vi "2-1.vi"(7 "kf(Hz/V)":dbl=50000.0, 8 "An(V)":dbl=0.02, 9 "带通Butterworth滤波器":cluster{"中心频率(Hz)":dbl, "带宽(Hz)":dbl}={"中心频率(Hz)"=150000.0, "带宽(Hz)"=220000.0}, 10 "调制信号":cluster{"fm(Hz)":dbl, "Am(V)":dbl}={"fm(Hz)"=5000.0, "Am(V)"=1.0}, 11 "载波信号":cluster{"fc(Hz)":dbl, "Ac(V)":dbl}={"fc(Hz)"=150000.0, "Ac(V)"=1.0}) -> (1 "频域":cluster{"f0":dbl, "df":dbl, "magnitude":dbl[]}(graph), 2 "时域 2":waveform(dbl)[](graph), 3 "时域":waveform(dbl)[](graph))   [LabVIEW 2018]
uses:
  <vilib>/Analysis/3filter.llb/Filter Passband Type.ctl
  <vilib>/Analysis/3filter.llb/Butterworth Filter (DBL).vi
  <vilib>/express/express analysis/Spectral/Block/exnSpectralBlock spectral measurements peak poly.vi
  <vilib>/express/express analysis/Spectral/Block/exnSpectralBlock spectral measurements peak WFM.vi
  <vilib>/express/express analysis/Spectral/XNode/ExpressSpectralMeasurementsBlockNode.xnode
  <vilib>/measure/NI_MABase.lvlib
  <vilib>/Analysis/NI_AALPro.lvlib
  <vilib>/Analysis/NI_AALBase.lvlib
panel:
  out "fh":dbl
  out "fl":dbl
  in  "选项卡控件":enum32{"调制", "滤波", "解调"}(tab)
  out "频域":cluster{"f0":dbl, "df":dbl, "magnitude":dbl[]}(graph)
  out "时域":waveform(dbl)(graph)
  out "卡森定则理论BT(Hz)":dbl
  out "数组":dbl[](array[numeric])
  out "调制信号":waveform(dbl)(graph)
  out "积分信号":waveform(dbl)(graph)
  out "采样参数（采样频率fs，采样数Ns）":cluster{dbl, dbl} {"?" format="%#_6f"; "?" format="%#_6f"}
  out "载波信号":waveform(dbl)(graph)
  # "采样率取1000*fc\n要显示n个周期的调制信号波形，\n则采样数Ns=n*fs/fm\nfh和fl为解调前滤波器\n的高和低截止频率"
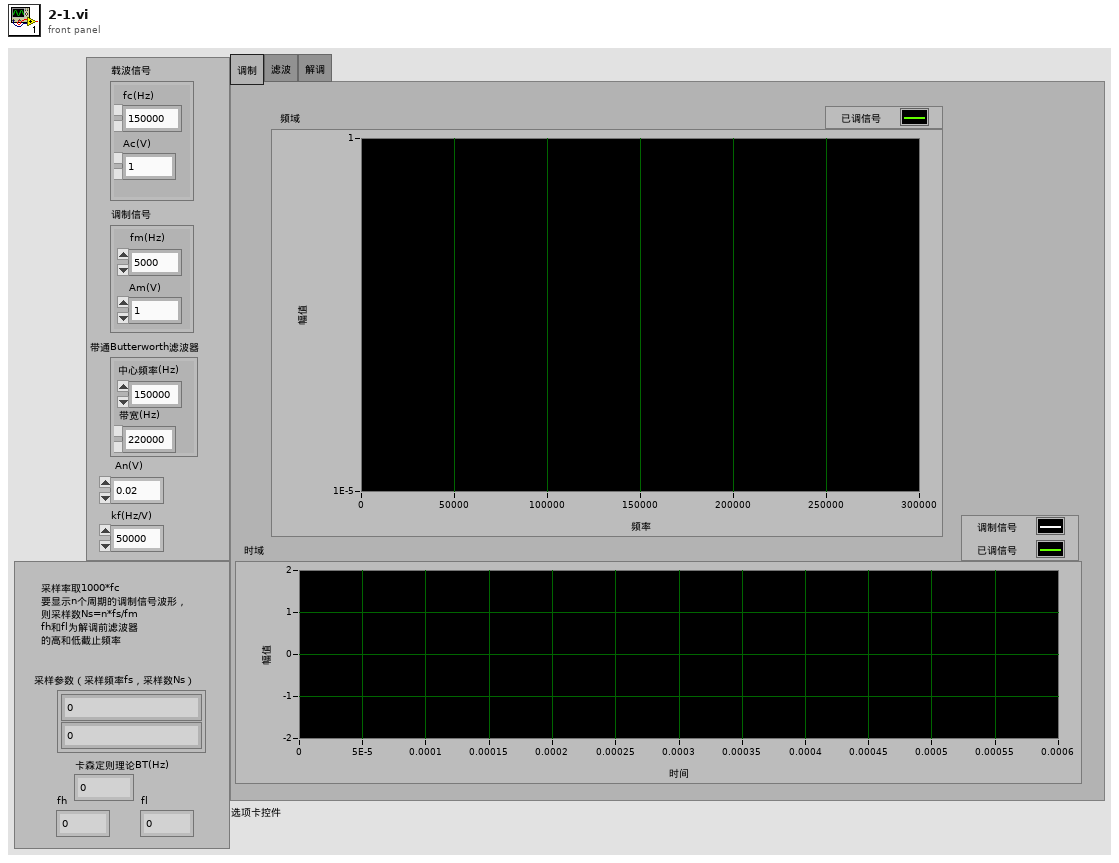
[diagram p1: front panel]
types:
  T1 = typedef "NI_AALBase.lvlib/Filter Passband Type.ctl" = enum32{"Lowpass", "Highpass", "Bandpass", "Bandstop"}
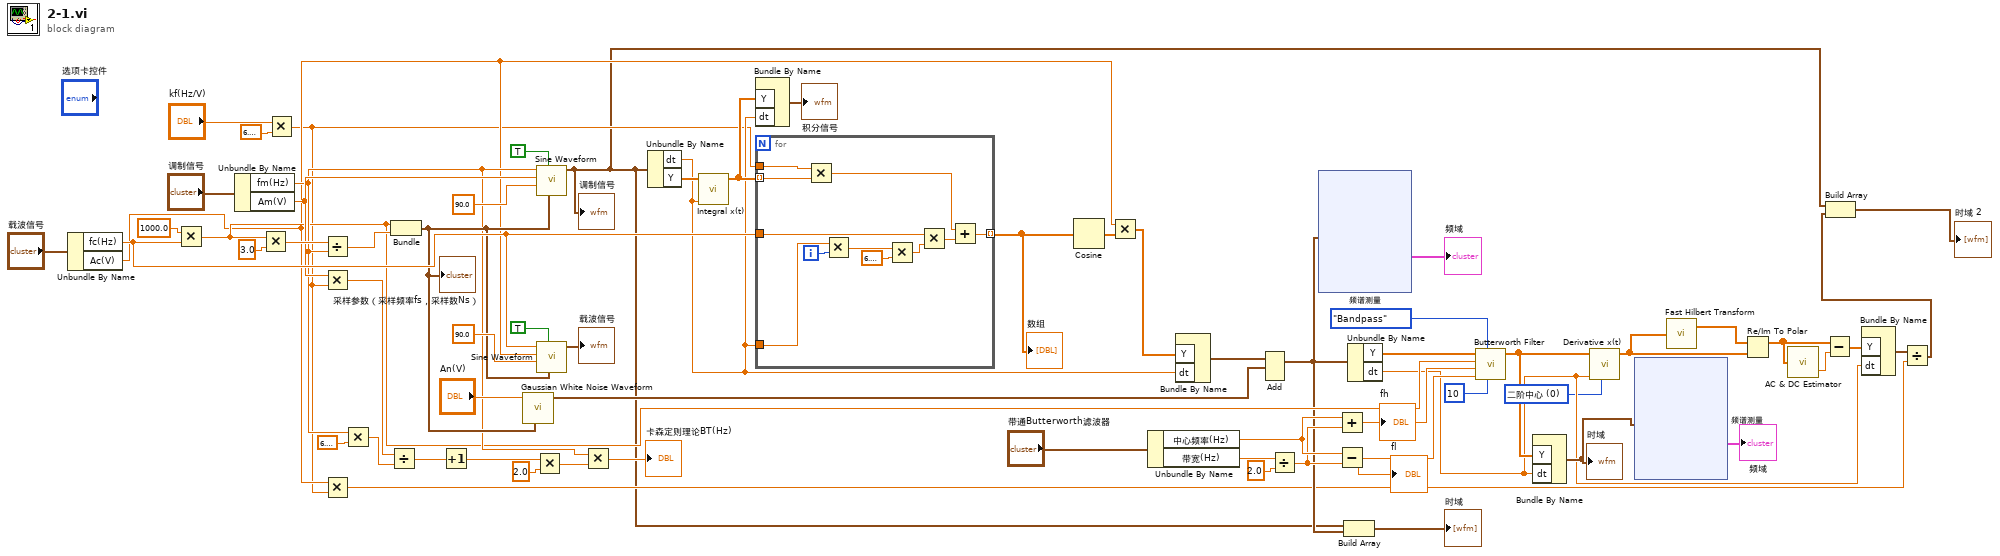
[diagram p0: block diagram]
diagram:
  w14 = u16 0 items=["二阶中心", "四阶中心", "前向", "后向"] ("method")
  n1 = Unbundle By Name("载波信号") -> ("fc(Hz)"=w53:dbl, "Ac(V)"=w10:dbl)
  n2 = Multiply(x=1000.0, y=w53) -> (x*y=w22:dbl)
  n3 = Unbundle By Name("调制信号") -> ("fm(Hz)"=w33:dbl, "Am(V)"=w40:dbl)
  n4 = Multiply(x=w22, y=3.0) -> (x*y=w61:dbl)
  n5 = Multiply(x="kf(Hz/V)", y=6.283185307179586) -> (x*y=w4:dbl)
  n6 = Divide(x=w61, y=w33) -> (x/y=w60:dbl)
  n7 = Multiply(x=w40, y=w4) -> (x*y=w38:dbl)
  n8 = Multiply(x=w10, y=w4) -> (x*y=w8:dbl)
  n9 = Multiply(x=w33, y=6.283185307179586) -> (x*y=w39:dbl)
  n10 = Divide(x=w38, y=w39) -> (x/y=w37:dbl)
  n11 = Bundle(w22, w60) -> (w47:cluster{dbl, dbl})  [unwired: 1 in]
  "采样参数（采样频率fs，采样数Ns）" <- w47
  n12 = Increment(x=w37) -> (x+1=w36:dbl)
  n13 = call <vilib>:"Gaussian White Noise Waveform.vi"("sampling info"=w47, "standard deviation"="An(V)") -> ("signal out"=w44:waveform(dbl))  [unwired: 8 in, 1 out]
  n14 = Multiply(x=w36, y=2.0) -> (x*y=w34:dbl)
  n15 = call <vilib>:"Sine Waveform.vi"("sampling info"=w47, "reset signal"=TRUE, "phase"=90.0, "amplitude"=w40, "frequency"=w33) -> ("signal out"=w2:waveform(dbl))  [unwired: 5 in, 1 out]
  "调制信号" <- w2
  n16 = call <vilib>:"Sine Waveform.vi"("sampling info"=w47, "reset signal"=TRUE, "phase"=90.0, "amplitude"=w10, "frequency"=w53) -> ("signal out"=→"载波信号":waveform(dbl))  [unwired: 5 in, 1 out]
  n17 = Multiply(x=w33, y=w34) -> (x*y=→"卡森定则理论BT(Hz)":dbl)
  n18 = Unbundle By Name(w2) -> ("dt"=w50:dbl, "Y"=w62:dbl[])
  n19 = call <vilib>:"Integral x(t).vi"("dt"=w50, "X"=w62) -> ("Integral X"=w54:dbl[])  [unwired: 8 in, 1 out]
  n20 = Bundle By Name("Y"=w54, "dt"=w50) -> (→"积分信号":waveform(dbl))  [unwired: 1 in]
  n21 = for {
    tunnel: w54 -> [w77] mode=indexing
    tunnel: w50 -> [w75]
    tunnel: w53 -> [w71]
    tunnel: [w68] -> w52 mode=indexing
    tunnel: w4 -> [w67]
    i -> [w76]
    n22 = Multiply(x=w67, y=w77) -> (x*y=w69:dbl)
    n23 = Multiply(x=w75, y=w76) -> (x*y=w73:dbl)
    n24 = Multiply(x=w73, y=6.283185307179586) -> (x*y=w72:dbl)
    n25 = Multiply(x=w71, y=w72) -> (x*y=w70:dbl)
    n26 = Add(x=w69, y=w70) -> (x+y=w68:dbl)
  }
  "数组" <- w52
  n27 = Cosine(x=w52) -> (cos(x)=w51:dbl[])
  n28 = Multiply(x=w10, y=w51) -> (x*y=w49:dbl[])
  n29 = Unbundle By Name("带通Butterworth滤波器") -> ("中心频率(Hz)"=w24:dbl, "带宽(Hz)"=w28:dbl)
  n30 = Bundle By Name("Y"=w49, "dt"=w50) -> (w46:waveform(dbl))  [unwired: 1 in]
  n31 = Add(1:w44, 2:w46) -> (0:w20:waveform(dbl))  [unwired: 1 in, 1 out]
  n32 = Divide(x=w28, y=2.0) -> (x/y=w23:dbl)
  n33 = xnode "频谱测量"("信号"=w20) -> ("FFT - （峰值）"=→"频域":cluster{"f0":dbl, "df":dbl, "magnitude":dbl[]})  [unwired: 1 in, 2 out]
  n34 = Add(x=w24, y=w23) -> (x+y=w26:dbl)
  "fh" <- w26
  n35 = Subtract(x=w24, y=w23) -> (x-y=w25:dbl)
  "fl" <- w25
  n36 = Build Array(w2, w20) -> (→"时域":waveform(dbl)[])
  n37 = Unbundle By Name(w20) -> ("Y"=w19:dbl[], "dt"=w15:dbl)
  n38 = call-poly <vilib>:"Butterworth Filter.vi"("order"=10, "filter type"=Filter_Passband_Type."Bandpass", "low cutoff freq: fl"=w25, "high cutoff freq: fh"=w26, "sampling freq: fs"=w22, "X"=w19) -> ("Filtered X"=w17:dbl[])  [unwired: 2 in, 1 out]
  n39 = Bundle By Name("Y"=w17, "dt"=w15) -> (w18:waveform(dbl))  [unwired: 1 in]
  "时域" <- w18
  n40 = call <vilib>:"Derivative x(t).vi"("method"=w14, "dt"=w15, "X"=w17) -> ("dX/dt"=w7:dbl[])  [unwired: 7 in, 1 out]
  n41 = xnode "频谱测量"("信号"=w18) -> ("FFT - （峰值）"=→"频域":cluster{"f0":dbl, "df":dbl, "magnitude":dbl[]})  [unwired: 1 in, 2 out]
  n42 = call <vilib>:"Fast Hilbert Transform.vi"("X"=w7) -> ("Hilbert{X}"=w16:dbl[])  [unwired: 1 out]
  n43 = Re/Im To Polar(2:w7, 3:w16) -> (1:w13:dbl[])  [unwired: 1 out]
  n44 = call <vilib>:"AC & DC Estimator.vi"("Signal (V)"=w13) -> ("DC estimate (V)"=w12:dbl)  [unwired: 1 out]
  n45 = Subtract(x=w13, y=w12) -> (x-y=w11:dbl[])
  n46 = Bundle By Name("Y"=w11, "dt"=w15) -> (w9:waveform(dbl))  [unwired: 1 in]
  n47 = Divide(x=w9, y=w8) -> (x/y=w3:waveform(dbl))
  n48 = Build Array(w2, w3) -> (→"时域 2":waveform(dbl)[])
